vi "Test Case.vi"(11 "Numeric":i32) -> (1 "Linha 2":string, 2 "Linha 1":string, 3 "Image Case":T1)   [LabVIEW 2016, in "MVP02 Custom Device.lvlib"]
uses:
  MVP02 Custom Device.lvlib
  Vision Case.ctl
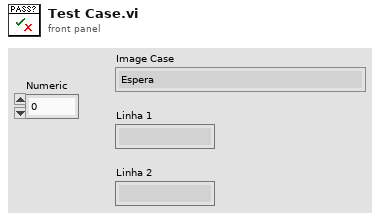
[diagram p1: front panel]
types:
  T1 = typedef "Vision Case.ctl" = enum16{"Espera", "OCR", "OCR2", "Outros"}
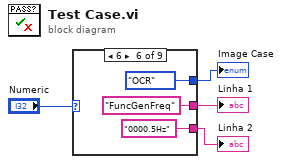
[diagram p0: block diagram]
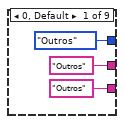
[diagram p2: hidden frame]
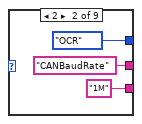
[diagram p3: hidden frame]
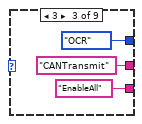
[diagram p4: hidden frame]
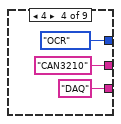
[diagram p5: hidden frame]
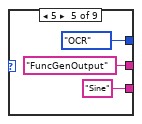
[diagram p6: hidden frame]
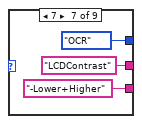
[diagram p7: hidden frame]
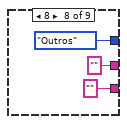
[diagram p8: hidden frame]
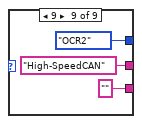
[diagram p9: hidden frame]
diagram:
  n1 = case shown="6" "Numeric" {
    tunnel: ["Outros" "CANBaudRate" "CANTransmit" ("String 2") "CAN3210" ("String 2") "FuncGenOutput" ("String 2") "FuncGenFreq" ("String 2") "LCDContrast" ("String 2") "" ("String 2") "High-SpeedCAN" ("String 2")] -> w3
    tunnel: ["Outros" "1M" "EnableAll" ("String") "DAQ" ("String") "Sine" ("String") "0000.5Hz" ("String") "-Lower+Higher" ("String") "" ("String") "" ("String")] -> w4
    tunnel: [Vision_Case."Outros" ("Image Case") Vision_Case."OCR" ("Image Case") Vision_Case."OCR" ("Image Case") Vision_Case."OCR" ("Image Case") Vision_Case."OCR" ("Image Case") Vision_Case."OCR" ("Image Case") Vision_Case."OCR" ("Image Case") Vision_Case."Outros" ("Image Case") Vision_Case."OCR2" ("Image Case")] -> w2
    frame 0, Default {
    }
    frame 2 {
    }
    frame 3 {
    }
    frame 4 {
    }
    frame 5 {
    }
    frame 6 {
    }
    frame 7 {
    }
    frame 8 {
    }
    frame 9 {
    }
  }
  "Linha 2" <- w4
  "Linha 1" <- w3
  "Image Case" <- w2
